vi "总氮启动(子VI).vi"(11 "参数":T2 {"站号" items=["总磷"=1, "总氮"=2, "氨氮"=3]}) -> (0 "error out":T1={"status"=FALSE, "代码"=4, "source"=""} caption="错误输出" {"代码" items=["执行成功"=1, "执行失败，但不知道原因"=2, "命令请求条件错误"=3, "通讯超时"=4, "系统繁忙不能执行"=5, "系统故障"=6, "没有数据"=100]})   [LabVIEW 2016]
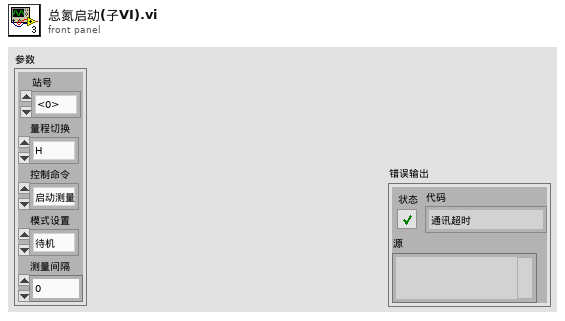
[diagram p1: front panel]
types:
  T1 = cluster{"status":bool, "代码":u16, "source":string}
  T2 = cluster{"站号":u16, "量程切换":enum32{"H", "L", "AUTO"}, "控制命令":enum16{"启动测量", "标样核查", "零点核查", "跨度核查", "空白测试", "平行样测试", "加标回收", "空白校准", "标样校准", "初始化（清洗）", "停止测试", "仪器重启", "校时", "模式设置", "测量间隔设置"}, "模式设置":enum16{"待机", "连续模式", "周期模式", "定点模式", "受控模式", "手动模式"}, "测量间隔":u16}
  T3 = enum16{"空闲", "水样测试", "标样核查", "零点核查", "跨度核查", "空白测试", "平行样测试", "加标回收", "空白校准", "标样校准", "初始化（清洗）"}
  T4 = cluster{"系统时间":timestamp, "工作状态":enum16{"空闲", "水样测试", "标样核查", "零点核查", "跨度核查", "空白测试", "平行样测试", "加标回收", "空白校准", "标样校准", "初始化（清洗）"}, "测量模式":enum16{"待机", "连续模式", "周期模式", "定点模式", "受控模式", "手动模式"}, "告警代码":u16, "故障代码":u16, "日志代码":u16, "软件版本":u16, "F0":sgl, "F1":sgl, "F2":sgl, "F3":sgl, "T":sgl, "H":sgl, "id":u16, "flowid":u16, "量程":u16, "总磷控温温度1":sgl, "营养盐控温温度2":sgl, "ADC":sgl}
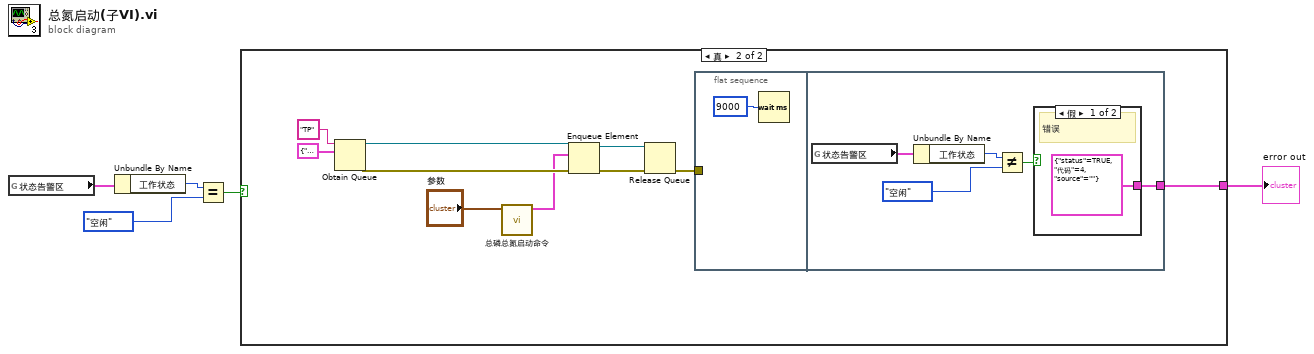
[diagram p0: block diagram]
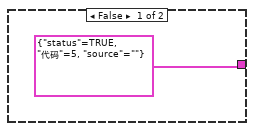
[diagram p2: hidden frame]
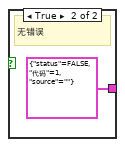
[diagram p3: hidden frame]
diagram:
  n1 = global read "VAR总磷总氮全局变量.vi" "状态告警区"() -> (w3:T4)
  n2 = Unbundle By Name(w3) -> ("工作状态"=w5:T3)
  n3 = Equal?(x=w5, y=T3."空闲") -> (x = y?=w2:bool)
  n4 = case shown="真" w2 {
    tunnel: [T1 {"status"=TRUE, "代码"=5, "source"=""} ("error out") w7] -> w1
    frame False {
    }
    frame True {
      n5 = Obtain Queue(name (unnamed)="TP" ("名称（未命名）"), element data type=cluster{"命令":string, "data":variant} {"命令"="", "data"=variant}) -> (queue out=w14:refnum<queue>, error out=w13:errorcluster)  [unwired: 3 in, 1 out]
      n6 = call "总磷总氮启动命令.vi"("参数"="参数") -> ("启动命令"=w11:cluster{"命令":string, "data":variant})  [unwired: 10 in]
      n7 = Enqueue Element(queue=w14, element=w11, error in (no error)=w13) -> (queue out=w10:refnum<queue>, error out=w9:errorcluster)  [unwired: 1 in, 1 out]
      n8 = Release Queue(queue=w10, error in (no error)=w9) -> (error out=w8:errorcluster)  [unwired: 1 in, 2 out]
      n9 = flat-sequence {
        tunnel: w8 -> [_]
        tunnel: [w22] -> w7
        frame #0 {
          n10 = Wait (ms)(milliseconds to wait=u32 9000 ("等待时间（毫秒）")) -> ()  [unwired: 1 out]
        }
        frame #1 {
          n11 = global read "VAR总磷总氮全局变量.vi" "状态告警区"() -> (w18:T4)
          n12 = Unbundle By Name(w18) -> ("工作状态"=w20:T3)
          n13 = Not Equal?(x=w20, y=T3."空闲") -> (x != y?=w19:bool)
          n14 = case shown="假" w19 {
            tunnel: [T1 {"status"=TRUE, "代码"=4, "source"=""} ("error out") T1 {"status"=FALSE, "代码"=1, "source"=""} ("error out")] -> w22
            frame False {
              # "错误"
            }
            frame True {
              # "无错误"
            }
          }
        }
      }
    }
  }
  "error out" <- w1
